vi "enumerateStaticDependencies.vi"(8 "error in (no error)":errorcluster, 11 "Measurement.IVCurve":refnum<class "Measurement.IVCurve.lvclass">) -> (0 "error out":errorcluster, 2 "Static Dependencies":refnum<class "Dependency.lvclass">[](array[class]), 3 "Measurement.IVCurve out":refnum<class "Measurement.IVCurve.lvclass">)   [LabVIEW 2017, in "Measurement.IVCurve.lvclass"]
doc: "JKI State Machine Objects (SMO) 1.3.0.56\nJKI - JKI\nCopyright (c) 2017, JKI"
uses:
  Measurement.IVCurve.lvclass
  <vilib>/JKI/JKI SMO/Dependency/Dependency.lvclass
  SMU/SMU.lvclass
  D:/Program Files (x86)/National Instruments/LabVIEW 2017/vi.lib/JKI/JKI SMO/SMO/SMO.lvclass
  Typedefs/Dependencies--Cluster.ctl
  Measurement/Measurement.lvclass
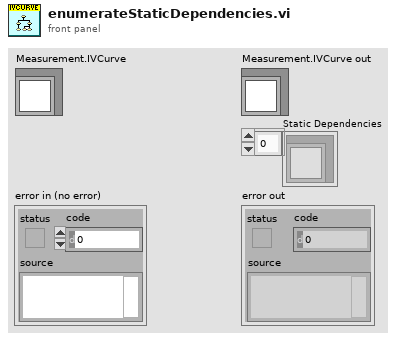
[diagram p1: front panel]
types:
  T1 = typedef "Measurement.IVCurve.lvclass/Dependencies--Cluster.ctl" = cluster{"SMU":refnum<class "SMU.lvclass">}
  T2 = typedef "Measurement.IVCurve.lvclass/Configuration--Cluster.ctl" = cluster{"Measurement.Type":T3, "Hardware":T4, "Measurement":T7}
  T3 = typedef "Measurement.lvclass/Measurement.Type--Enum.ctl" = enum16{"Free", "I/V Curve", "Wavelength sweeping", "Photocurrent mapping"}
  T4 = typedef "Measurement.IVCurve.lvclass/Configuration.Hardware--Cluster.ctl" = cluster{"SMU":T5}
  T5 = typedef "Measurement.lvclass/Configuration.SMU--Cluster.ctl" = cluster{"Enable":bool, "SMU Model":string, "Configuration":T6}
  T6 = typedef "SMU.lvclass/Configuration--Cluster.ctl" = cluster{"VISA Resource":string, "Channel":string}
  T7 = typedef "Measurement.IVCurve.lvclass/Configuration.Measurement--Cluster.ctl" = cluster{"SMU Voltage Start, V":dbl, "SMU Voltage Stop, V":dbl, "SMU Voltage Step, V":dbl, "Delay time, ms":u16, "Accumulation":u16}
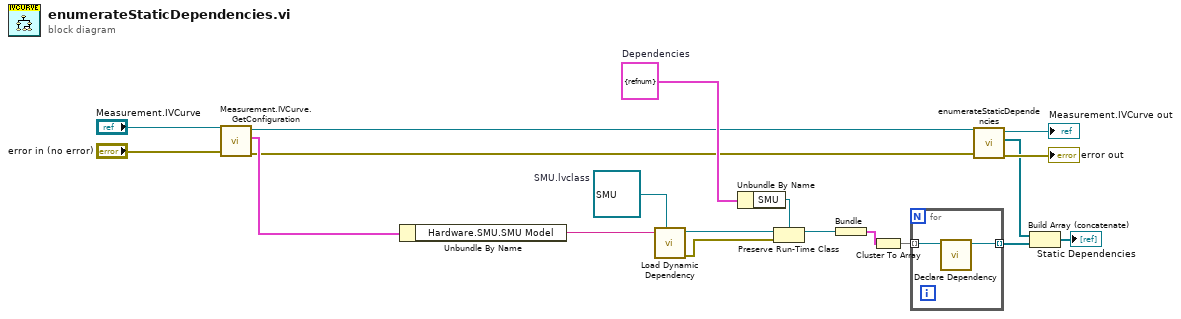
[diagram p0: block diagram]
diagram:
  w6 = T1 {"SMU"=refnum}  # Dependencies
  w16 = refnum<class "SMU.lvclass"> refnum  # SMU.lvclass
  n1 = call "Measurement.IVCurve.GetConfiguration.vi"("error in (no error)"="error in (no error)", "Measurement.IVCurve"="Measurement.IVCurve") -> ("error out"=w4:errorcluster, "Configuration"=w7:T2, "Measurement.IVCurve out"=w5:refnum<class "Measurement.IVCurve.lvclass">)  [unwired: 7 in]
  n2 = Unbundle By Name(w7) -> ("Hardware.SMU.SMU Model"=w17:string)
  n3 = call "Load Dynamic Dependency.vi"("SMO in"=w16, "Class Name"=w17) -> ("error out"=w13:errorcluster, "SMO out"=w14:refnum<class "SMU.lvclass">)  [unwired: 8 in]
  n4 = Unbundle By Name(w6) -> ("SMU"=w15:refnum<class "SMU.lvclass">)
  n5 = Preserve Run-Time Class(object in=w14, error in=w13, 2:w15) -> (object out=w12:refnum<class "SMU.lvclass">)  [unwired: 1 out]
  n6 = Bundle("SMU"=w12) -> (w11:cluster{"SMU":refnum<class "SMU.lvclass">})  [unwired: 1 in]
  n7 = Cluster To Array(cluster=w11) -> (array=w10:refnum<class "SMU.lvclass">[])
  n8 = for {
    tunnel: [w21] -> w3 mode=indexing
    tunnel: w10 -> [w20] mode=indexing
    n9 = call <vilib>:"Declare Dependency.vi"("Type"=w20) -> ("Dependency out"=w21:refnum<class "Dependency.lvclass">)  [unwired: 9 in, 1 out]
  }
  n10 = call-parent "enumerateStaticDependencies.vi"("error in (no error)"=w4, "SMO"=w5) -> ("error out"=→"error out":errorcluster, "Static Dependencies"=w2:refnum<class "Dependency.lvclass">[], "SMO out"=→"Measurement.IVCurve out":refnum<class "Measurement.IVCurve.lvclass">)  [unwired: 7 in]
  n11 = Build Array (concatenate)(w2, w3) -> (→"Static Dependencies":refnum<class "Dependency.lvclass">[])
